vi "Handle Configuration Updated.vi"(8 "error in (no error)":errorcluster, 10 "Name":string, 11 "New Data":variant) -> (0 "error out":errorcluster, 2 "Addressed to this Module":bool, 3 "Latest Data":T1)   [LabVIEW 2020, in "Performance Monitor UI.lvlib" / "Configuration.lvlib"]
doc: "Handles the DCFG Framework Broadcast Event \"Configuration Updated\". Place this VI in your DQMH_EVENT_MAIN event structure in the DQMH Module Main.vi where this configuration will be used.\nThis event fires when the configuration is updated via any of the pages for this library.\n\nThis VI updates the global that stores the configuration that is accessed by other parts of the module.\n_____\nBased on DCFG Project Template 1.0.0.21.\n____\nPeloton Config 1.0.0.2\nCopyright (c) 2022, Peloton"
uses:
  Configuration.lvlib
  Configuration--cluster.ctl
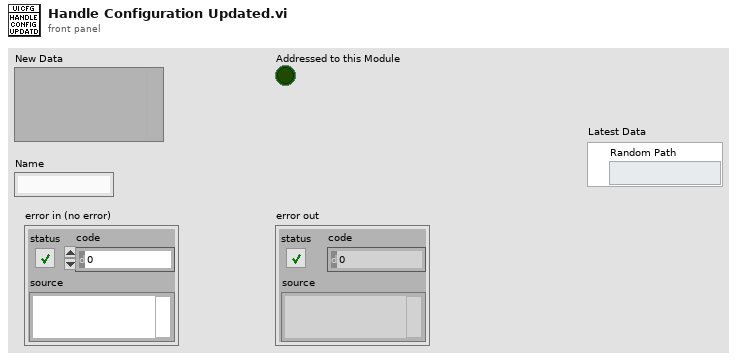
[diagram p1: front panel]
types:
  T1 = typedef "Performance Monitor UI.lvlib/Configuration.lvlib/Configuration--cluster.ctl" = cluster{"Random Path":path}
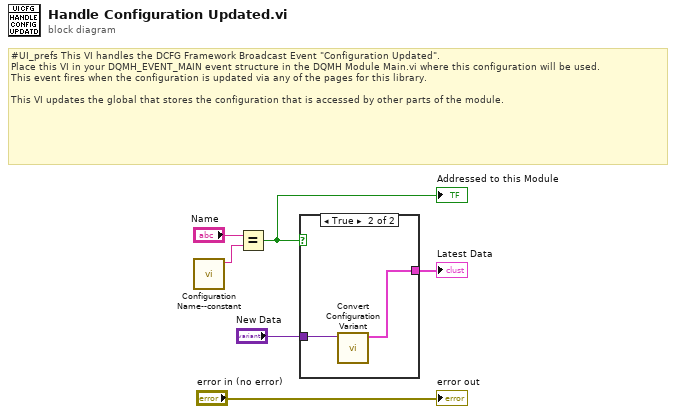
[diagram p0: block diagram]
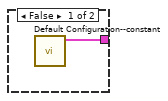
[diagram p2: hidden frame]
diagram:
  # "#UI_prefs This VI handles the DCFG Framework Broadcast Event \"Configuration Updated\".\nPlace this VI in your DQMH_EVENT_MAIN event structure in the DQMH Module Main.vi where this configuration will be used.\nThis event fires when the configuration is updated via any of the pages for this library.\n \nThis VI updates the global that stores the configuration that is accessed by other parts of the module."
  n1 = call "Configuration Name--constant.vi"() -> ("Configuration Name"=w3:string)  [unwired: 11 in]
  n2 = Equal?(x="Name", y=w3) -> (x = y?=w4:bool)
  "Addressed to this Module" <- w4
  n3 = case shown="True" w4 {
    tunnel: "New Data" -> [_ w9]
    tunnel: [w7 w8] -> w2
    frame False {
      n4 = call "Default Configuration--constant.vi"() -> ("Default Configuration"=w7:T1)  [unwired: 11 in]
    }
    frame True {
      n5 = call "Convert Configuration Variant.vi"("Current Configuration"=w9) -> ("Configuration"=w8:T1)  [unwired: 8 in, 2 out]
    }
  }
  "Latest Data" <- w2
  "error out" <- "error in (no error)"
